vi "Update Subpanel.vi"(8 "error in":errorcluster, 10 "sPanel":i32, 11 "GUI Facade in":refnum<class "GUI Facade.lvclass">) -> (0 "error out":errorcluster, 3 "GUI Facade out":refnum<class "GUI Facade.lvclass">)   [LabVIEW 2018, in "GUI Facade.lvclass"]
doc: "Removes the current VI in the subpanel and inserts the one requested into the subpanel."
uses:
  GUI Facade.lvclass
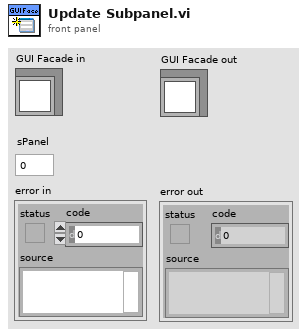
[diagram p1: front panel]
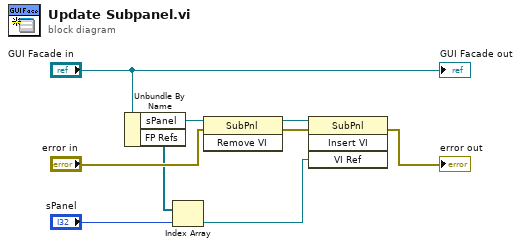
[diagram p0: block diagram]
diagram:
  n1 = Unbundle By Name("GUI Facade in") -> ("sPanel"=w5:refnum<vi>, "FP Refs"=w2:refnum<vi>[])
  n2 = Index Array(array=w2, index="sPanel") -> (element=w1:refnum<vi>)
  n3 = invoke class="SubPnl" method="Remove VI"(reference=w5, error in="error in") -> (reference out=w3:refnum<vi>, error out=w4:errorcluster)  [unwired: 1 in, 1 out]
  n4 = invoke class="SubPnl" method="Insert VI"(reference=w3, error in=w4, "VI Ref"=w1) -> (error out=→"error out":errorcluster)  [unwired: 1 in, 3 out]
  "GUI Facade out" <- "GUI Facade in"
